vi "SR830SetDCOffset.vi"(5 "Step dwell time (ms)":u32=50, 7 "Voltage Step (V)":dbl=0.001, 8 "error in (no error)":errorcluster, 9 "Target Voltage (V)":dbl, 10 "Aux Channel (1: Channel 1)":u16(ring)=2 items=["Channel 1"=1, "Channel 2"=2, "Channel 3"=3, "Channel 4"=4], 11 "VISA resource name":refnum<visa-resource-name>="SR830LockIn2") -> (0 "error out":errorcluster, 1 "Final Voltage (V)":dbl=0.016400000000000192, 2 "Start Voltage (V)":dbl=-1.0335999999999999, 3 "VISA resource name out":refnum<visa-resource-name>="SR830LockIn2")   [LabVIEW 2016]
uses:
  <instrlib>/Stanford Research 830/Stanford Research 830.lvlib
panel:
  # "This VI uses the Aux Out of the SR830 to control the DC Offset for AC+DC.\nChoose either Aux Out 1 or Aux out 2 as the control channel\nDefault to Aux Out 2 because Aux Out 1 is default to control magnetic field\nMAKE SURE TO USE ISOLATION TRANSFORMER"
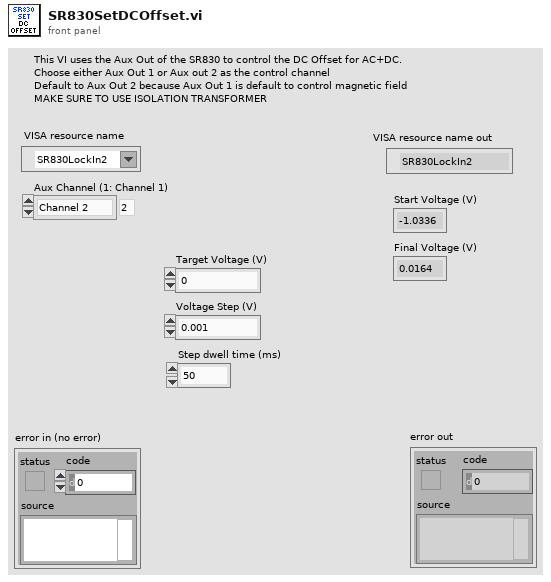
[diagram p1: front panel]
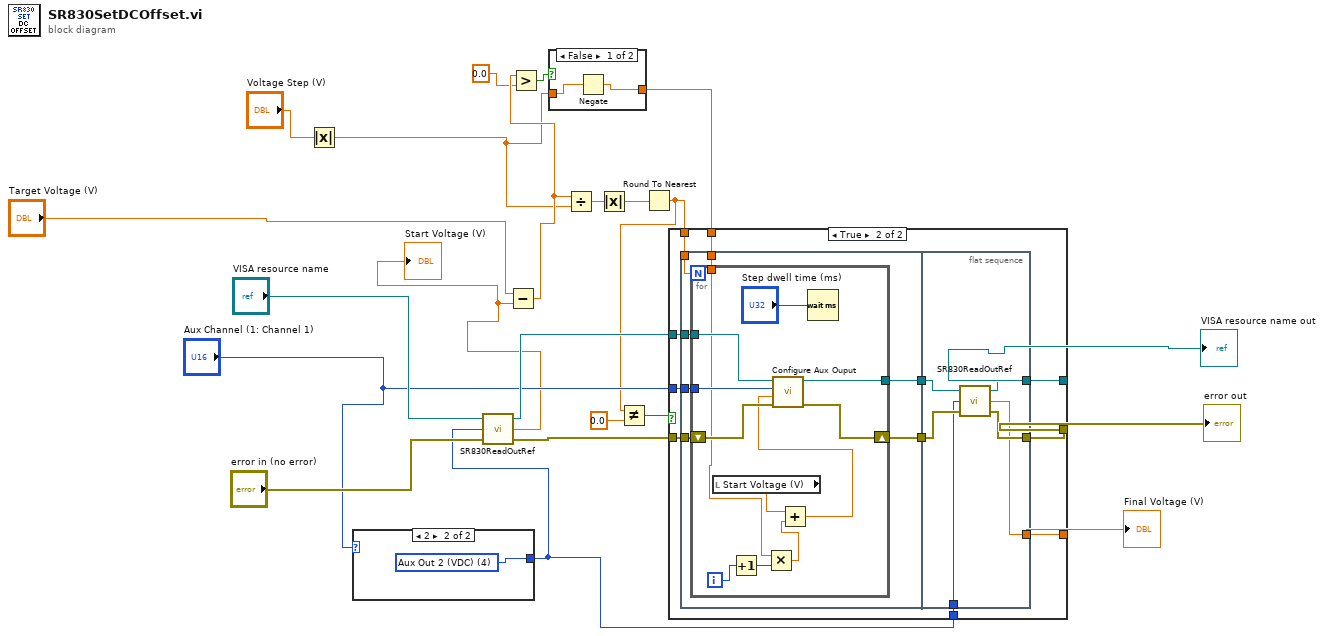
[diagram p0: block diagram]
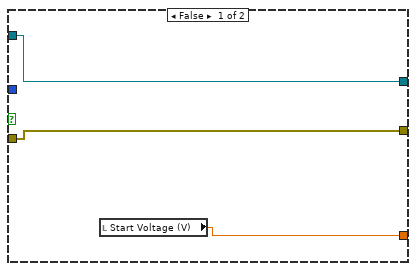
[diagram p3: hidden frame]
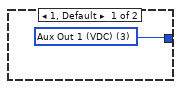
[diagram p4: hidden frame]
diagram:
  n1 = Absolute Value(x="Voltage Step (V)") -> (abs(x)=w8:dbl)
  n2 = case shown="2" "Aux Channel (1: Channel 1)" {
    tunnel: [w23 w24] -> w1
    frame 1, Default {
      w23 = u16 3 items=["Voltage Out (Vrms)"=1, "Frequency (Hz)"=2, "Aux Out 1 (VDC)"=3, "Aux Out 2 (VDC)"=4, "Time Constant (s)"=5] ("ReadOut (1: Voltage Amplitude)")
    }
    frame 2 {
      w24 = u16 4 items=["Voltage Out (Vrms)"=1, "Frequency (Hz)"=2, "Aux Out 1 (VDC)"=3, "Aux Out 2 (VDC)"=4, "Time Constant (s)"=5, "Roll-Off Slope (dB/oct)"=6] ("ReadOut (1: Voltage Amplitude)")
    }
  }
  n3 = call "SR830ReadOutRef.vi"("error in (no error)"="error in (no error)", "ReadOut (1: Voltage Amplitude)"=w1, "VISA resource name"="VISA resource name") -> ("error out"=w19:errorcluster, "ReadOut"=w2:dbl, "VISA resource name out"=w20:refnum<visa-resource-name>)
  "Start Voltage (V)" <- w2
  n4 = Subtract(x="Target Voltage (V)", y=w2) -> (x-y=w11:dbl)
  n5 = Greater?(x=w11, y=0.0) -> (0:w9:bool)
  n6 = case shown="False" w9 {
    tunnel: w8 -> [w26 w27]
    tunnel: [w25 w27] -> w7
    frame False {
      n7 = Negate(x=w26) -> (-x=w25:dbl)
    }
    frame True {
    }
  }
  n8 = Divide(x=w11, y=w8) -> (x/y=w16:dbl)
  n9 = Absolute Value(x=w16) -> (abs(x)=w15:dbl)
  n10 = Round To Nearest(number=w15) -> (nearest integer value=w12:dbl)
  n11 = Not Equal?(x=w12, y=0.0) -> (x != y?=w14:bool)
  n12 = case shown="True" w14 {
    tunnel: [w30 w41] -> w4
    tunnel: [w29 w40] -> w3
    tunnel: w20 -> [w30 w39]
    tunnel: w19 -> [w29 w38]
    tunnel: "Aux Channel (1: Channel 1)" -> [_ w37]
    tunnel: w12 -> [_ w36]
    tunnel: w7 -> [_ w35]
    tunnel: [w28 w34] -> w6
    tunnel: w1 -> [_ w31]
    frame False {
      n13 = local read "Start Voltage (V)"() -> (w28:dbl)
    }
    frame True {
      n14 = flat-sequence {
        tunnel: w39 -> [w46]
        tunnel: w38 -> [w45]
        tunnel: w37 -> [w44]
        tunnel: w36 -> [w43]
        tunnel: w35 -> [w42]
        tunnel: [w48] -> w33
        tunnel: [w47] -> w32
        tunnel: [w62] -> w34
        tunnel: [w64] -> w40
        tunnel: [w63] -> w41
        tunnel: w33 -> [w66]
        tunnel: w32 -> [w65]
        tunnel: w31 -> [w61]
        frame #0 {
          n15 = for {
            N: w43 -> [_]
            tunnel: w44 -> [w60]
            shift-right: [w56] -> w47
            shift-left: w45 -> [w58]
            tunnel: w46 -> [w59]
            tunnel: [w57] -> w48
            tunnel: w42 -> [w52]
            i -> [w55]
            n16 = local read "Start Voltage (V)"() -> (w54:dbl)
            n17 = Increment(x=w55) -> (x+1=w53:i32)
            n18 = Multiply(x=w52, y=w53) -> (x*y=w51:dbl)
            n19 = Add(x=w54, y=w51) -> (x+y=w49:dbl)
            n20 = call <instrlib>:"Configure Aux Ouput.vi"("error in (no error)"=w58, "Aux Output Voltage (1 V)"=w49, "Aux Channel (1: Channel 1)"=w60, "VISA resource name"=w59) -> ("error out"=w56:errorcluster, "VISA resource name out"=w57:refnum<visa-resource-name>)  [unwired: 6 in]
            n21 = Wait (ms)(milliseconds to wait="Step dwell time (ms)") -> ()  [unwired: 1 out]
          }
        }
        frame #1 {
          n22 = call "SR830ReadOutRef.vi"("error in (no error)"=w65, "ReadOut (1: Voltage Amplitude)"=w61, "VISA resource name"=w66) -> ("error out"=w64:errorcluster, "ReadOut"=w62:dbl, "VISA resource name out"=w63:refnum<visa-resource-name>)
        }
      }
    }
  }
  "VISA resource name out" <- w4
  "error out" <- w3
  "Final Voltage (V)" <- w6
